vi "design pattern-sol1-prac.vi"() -> ()   [LabVIEW 2013]
panel:
  in  "Tank Control":dbl(slide) scale=0.0..10.0
  out "Task 1":dbl(slide) scale=0.0..10.0
  out "Task 2":dbl(slide) scale=0.0..10.0
  in  "stop":bool
  in  "OK Button":bool
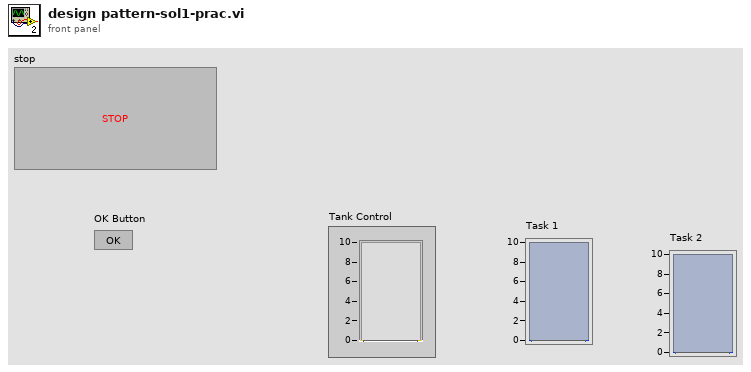
[diagram p1: front panel]
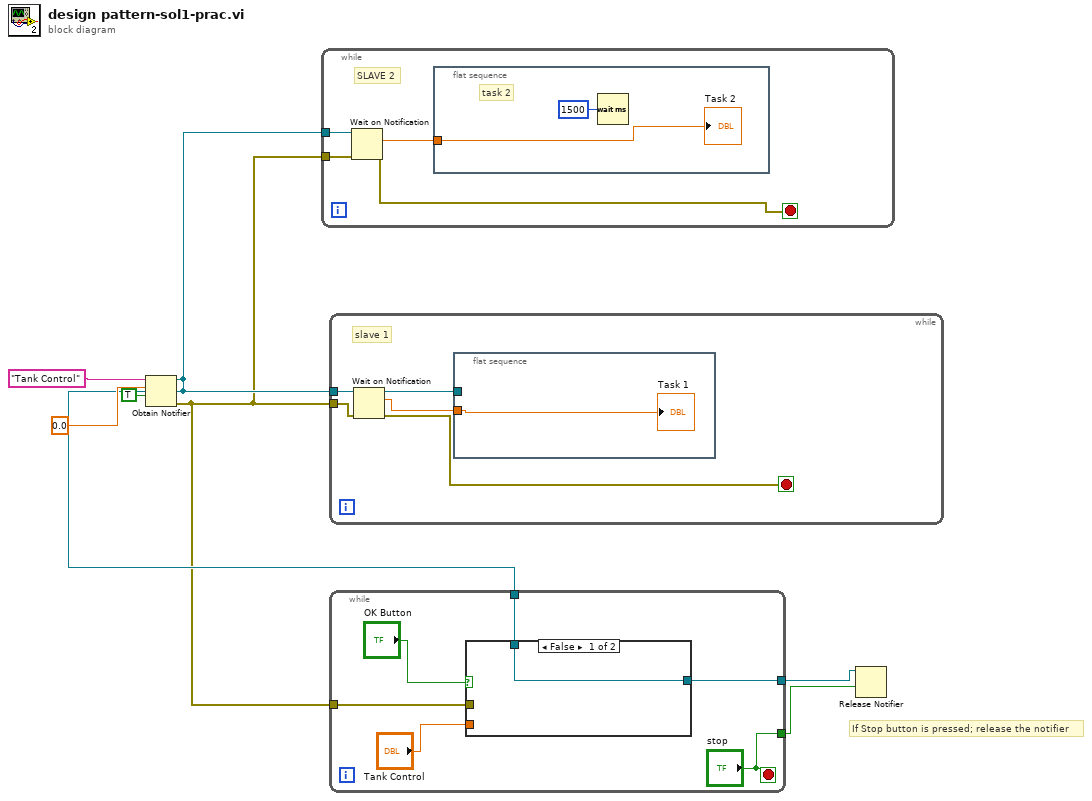
[diagram p0: block diagram]
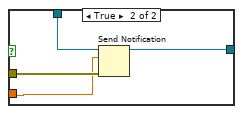
[diagram p2: hidden frame]
diagram:
  # "If Stop button is pressed; release the notifier"
  n1 = Obtain Notifier(name (unnamed)="Tank Control", notification data type=0.0, create if not found? (T)=TRUE) -> (notifier out=w4:refnum<notifier>, error out=w3:errorcluster)  [unwired: 1 in, 1 out]
  n2 = while {
    tunnel: w4 -> [w11]
    tunnel: w3 -> [w10]
    stop <- w9 stop-if-true
    # "SLAVE 2"
    n3 = Wait on Notification(notifier=w11, error in (no error)=w10) -> (notification=w8:dbl, error out=w9:errorcluster)  [unwired: 2 in, 2 out]
    n4 = flat-sequence {
      tunnel: w8 -> [w12]
      frame #0 {
        # "task 2"
        n5 = Wait (ms)(milliseconds to wait=u32 1500) -> ()  [unwired: 1 out]
        "Task 2" <- w12
      }
    }
  }
  n6 = while {
    tunnel: w4 -> [w18]
    tunnel: w3 -> [w17]
    stop <- w15 stop-if-true
    # "slave 1"
    n7 = Wait on Notification(notifier=w18, error in (no error)=w17) -> (notifier out=w16:refnum<notifier>, notification=w14:dbl, error out=w15:errorcluster)  [unwired: 2 in, 1 out]
    n8 = flat-sequence {
      tunnel: w16 -> [_]
      tunnel: w14 -> [w19]
      frame #0 {
        "Task 1" <- w19
      }
    }
  }
  n9 = while {
    tunnel: w4 -> [w24]
    tunnel: w3 -> [w23]
    tunnel: [w22] -> w2
    tunnel: ["stop"] -> w1
    stop <- "stop" stop-if-true
    n10 = case shown="False" "OK Button" {
      tunnel: w24 -> [w26 w30]
      tunnel: w23 -> [_ w29]
      tunnel: [w26 w28] -> w22
      tunnel: "Tank Control" -> [_ w27]
      frame False {
      }
      frame True {
        n11 = Send Notification(notification=w27, notifier=w30, error in (no error)=w29) -> (notifier out=w28:refnum<notifier>)  [unwired: 1 out]
      }
    }
  }
  n12 = Release Notifier(notifier=w2, force destroy? (F)=w1) -> ()  [unwired: 1 in, 3 out]
